vi "Cal Fov.vi"(2 "min":dbl format="%.2f", 3 "Span":dbl format="%.2f") -> (0 "min":dbl[](array[numeric]) format="%.2f", 1 "Span":dbl[](array[numeric]) format="%.2f")   [LabVIEW 2016]
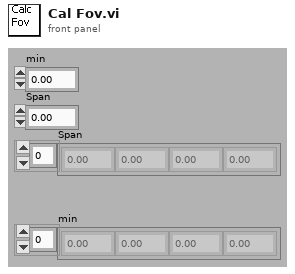
[diagram p1: front panel]
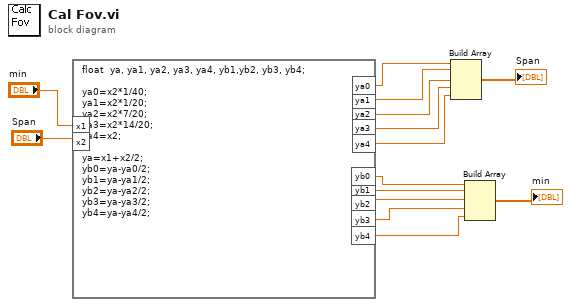
[diagram p0: block diagram]
diagram:
  n1 = formula code="float  ya, ya1, ya2, ya3, ya4, yb1,yb2, yb3, yb4; \n\nya0=x2*1/40;\nya1=x2*1/20;\nya2=x2*7/20;\nya3=x2*14/20;\nya4=x2;\n\nya=x1+x2/2;\nyb0=ya-ya0/2;\nyb1=ya-ya1/2;\nyb2=ya-ya2/2;\nyb3=ya-ya3/2;\nyb4=ya-ya4/2;"("x1"="min", "x2"="Span") -> ("ya2"=w13:dbl, "ya1"=w14:dbl, "ya3"=w12:dbl, "yb1"=w11:dbl, "yb2"=w10:dbl, "yb3"=w9:dbl, "ya4"=w4:dbl, "yb4"=w3:dbl, "ya0"=w2:dbl, "yb0"=w1:dbl)
  n2 = Build Array(w2, w14, w13, w12, w4) -> (→"Span":dbl[])
  n3 = Build Array(w1, w11, w10, w9, w3) -> (→"min":dbl[])
